vi "Plot menu activation.vi"(7 "BluePlotHandle in":refnum<class "RocketPlotHandle.lvclass">, 8 "error in (no error)":errorcluster, 9 "Coords":T4, 10 "Refs":T5, 11 "MenuRef":refnum<k9>) -> (0 "error out":errorcluster, 1 "Location":T1, 2 "Discard?":bool, 3 "MenuRef":refnum<k9>)   [LabVIEW 2021, in "RocketPlot.lvlib"]
uses:
  RocketPlot.lvlib
  Classes/RocketPlotHandle/RocketPlotHandle.lvclass
  TypeDefs/Plot UI references.ctl
  <userlib>/bjustice/TipStripOOPanel/Classes/TipPanelHandle/TipPanelHandle.lvclass
  TypeDefs/Plot top row.ctl
  <vilib>/Utility/miscctls.llb/LVPoint32TypeDef.ctl
  TypeDefs/Shortcut Location.ctl
  Plot menu activation submenu type v2.ctl
  TypeDefs/Plot axis.ctl
  Plot scale refnum to LUT name.vi
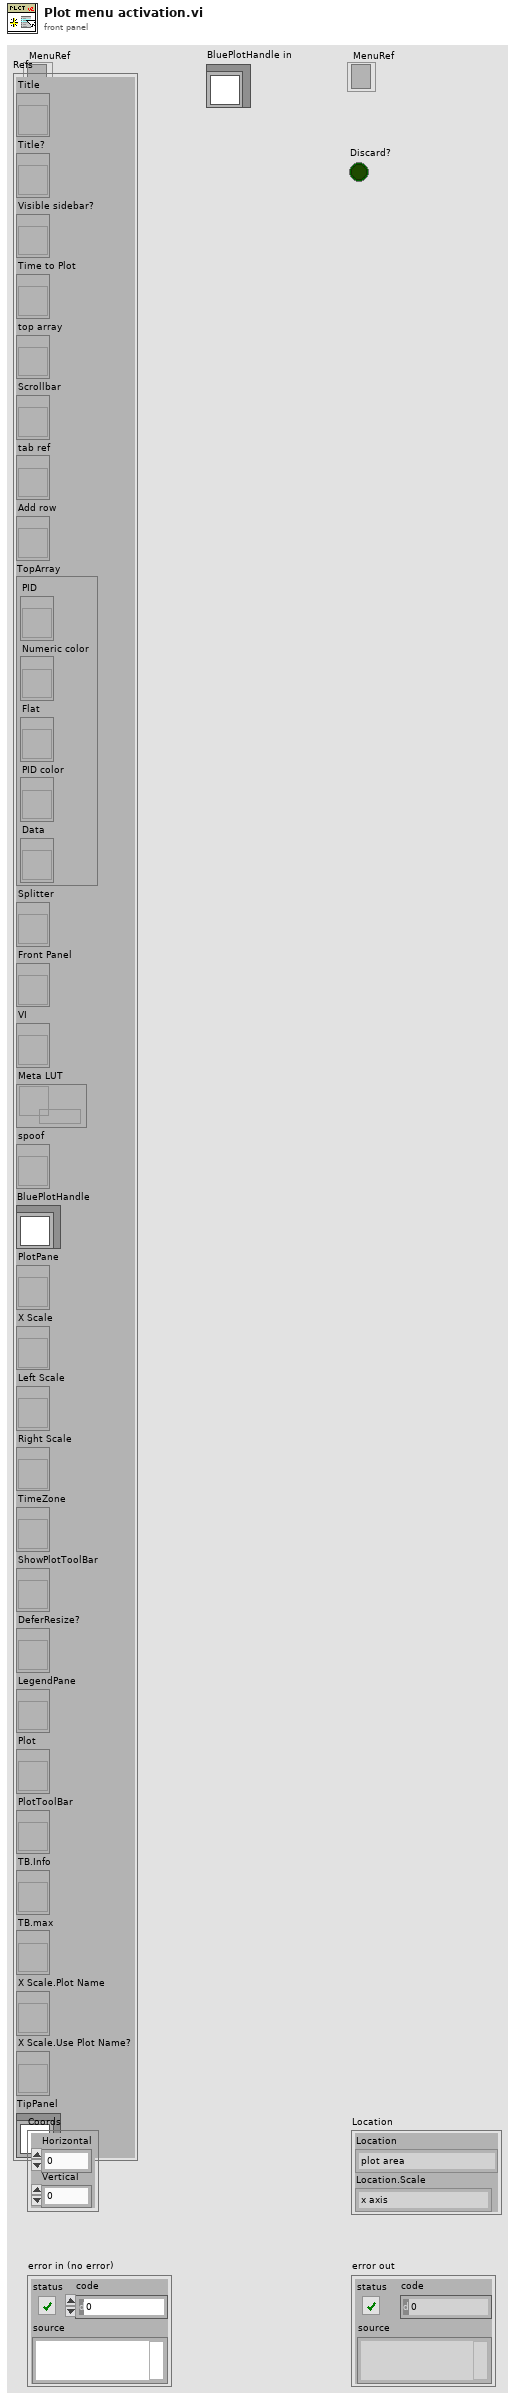
[diagram p1: front panel]
types:
  T1 = typedef "RocketPlot.lvlib/Shortcut Location.ctl" = cluster{"Location":T2, "Location.Scale":T3}
  T2 = typedef "RocketPlot.lvlib/Plot menu activation submenu type v2.ctl" = enum16{"plot area", "plot border", "markers", "scale"}
  T3 = typedef "RocketPlot.lvlib/Plot axis.ctl" = enum16{"x axis", "left axis", "right axis"}
  T4 = typedef "LVPoint32TypeDef.ctl" = cluster{"Horizontal":i32, "Vertical":i32}
  T5 = typedef "RocketPlot.lvlib/Plot UI references.ctl" = cluster{"Title":refnum<vi>, "Title?":refnum<vi>, "Visible sidebar?":refnum<vi>, "Time to Plot":refnum<vi>, "top array":refnum<vi>, "Scrollbar":refnum<vi>, "tab ref":refnum<vi>, "Add row":refnum<vi>, "TopArray":cluster{"PID":refnum<vi>, "Numeric color":refnum<vi>, "Flat":refnum<vi>, "PID color":refnum<vi>, "Data":refnum<vi>}, "Splitter":refnum<vi>, "Front Panel":refnum<vi>, "VI":refnum<vi>, "Meta LUT":refnum<data-value>, "spoof":refnum<vi>, "BluePlotHandle":refnum<class "RocketPlotHandle.lvclass">, "PlotPane":refnum<vi>, "X Scale":refnum<vi>, "Left Scale":refnum<vi>, "Right Scale":refnum<vi>, "TimeZone":refnum<vi>, "ShowPlotToolBar":refnum<vi>, "DeferResize?":refnum<vi>, "LegendPane":refnum<vi>, "Plot":refnum<vi>, "PlotToolBar":refnum<vi>, "TB.Info":refnum<vi>, "TB.max":refnum<vi>, "X Scale.Plot Name":refnum<vi>, "X Scale.Use Plot Name?":refnum<vi>, "TipPanel":refnum<class "TipPanelHandle.lvclass">}
  T6 = typedef "RocketPlot.lvlib/PlatMods.ctl" = cluster{"Shift":bool, "Ctrl":bool, "Alt":bool}
  T7 = typedef "RocketPlot.lvlib/Plot scale meta JSON.ctl" = cluster{"Type":T3, "Grid Colors:Major Color":u32, "Grid Colors:Minor Color":u32, "Style":u8, "Tick Colors:Tick Color":u32, "Tick Colors:Minor Tick Color":u32, "Format String":string, "State":T8, "AxisFocus":refnum<vi>}
  T8 = typedef "RocketPlot.lvlib/Plot scale meta state.ctl" = cluster{"Visible":bool, "Focus":bool, "Multi-Y":bool}
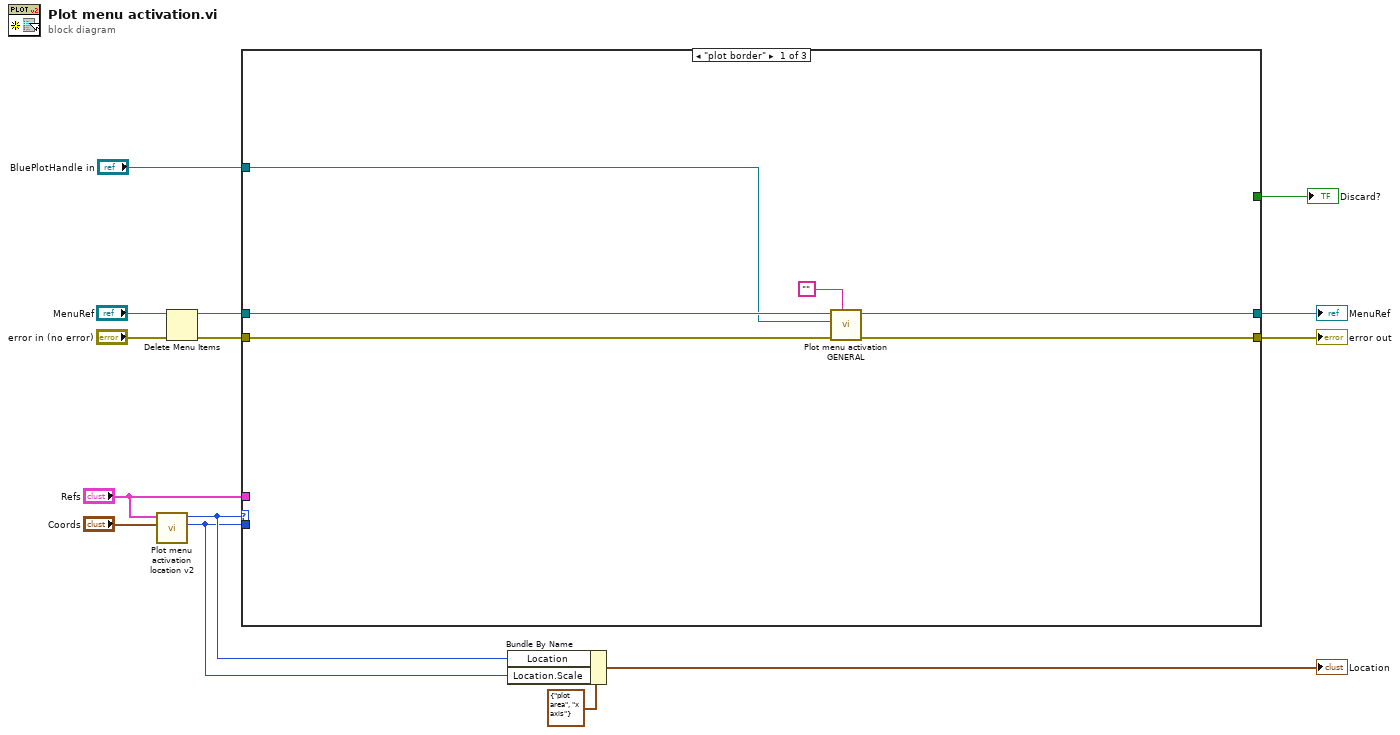
[diagram p0: block diagram]
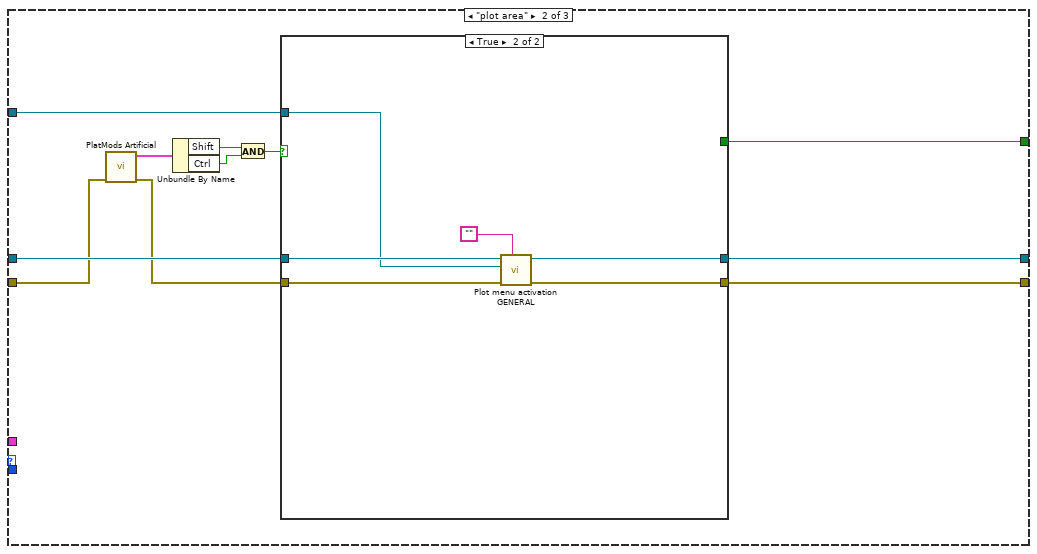
[diagram p2: hidden frame]
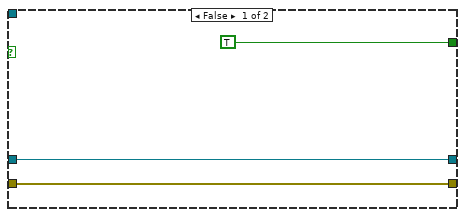
[diagram p3: hidden frame]
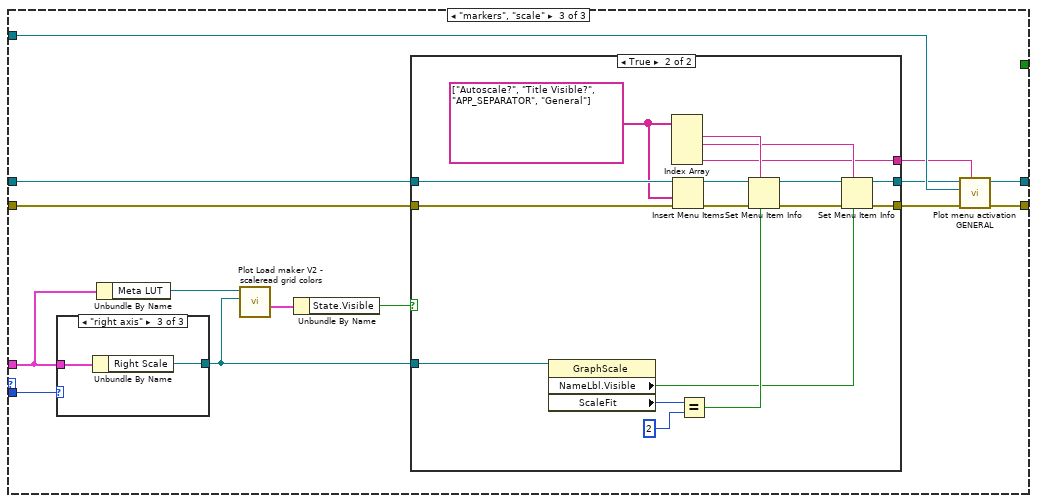
[diagram p4: hidden frame]
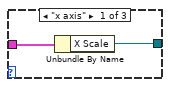
[diagram p6: hidden frame]
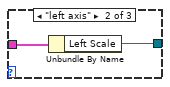
[diagram p7: hidden frame]
diagram:
  n1 = call "Plot menu activation location v2.vi"("Coords"="Coords", "Refs"="Refs") -> ("Location.Scale"=w3:T3, "Location"=w4:T2)  [unwired: 7 in, 1 out]
  n2 = Delete Menu Items(6:"error in (no error)", 9:"MenuRef") -> (0:w9:errorcluster, 3:w10:refnum<k9>)  [unwired: 2 in]
  n3 = case shown="\"plot border\"" w4 {
    tunnel: w3 -> [_ _ w54]
    tunnel: "Refs" -> [_ _ w45]
    tunnel: w10 -> [w18 w30 w53]
    tunnel: w9 -> [w20 w25 w52]
    tunnel: [w19 w31 w50] -> w8
    tunnel: "BluePlotHandle in" -> [w17 w29 w49]
    tunnel: [w15 w28 w46] -> w6
    tunnel: [_ w26 _] -> w1
    frame "plot border" {
      n4 = call "Plot menu activation GENERAL.vi"("menu tag"="", "error in (no error)"=w20, "BluePlotHandle in"=w17, "MenuRef"=w18) -> ("error out"=w19:errorcluster, "MenuRef"=w15:refnum<k9>)  [unwired: 6 in]
    }
    frame "plot area" {
      n5 = call "PlatMods Artificial.vi"("error in (no error)"=w25) -> ("error out"=w24:errorcluster, "PlatMods"=w27:T6)  [unwired: 9 in]
      n6 = Unbundle By Name(w27) -> ("Shift"=w23:bool, "Ctrl"=w22:bool)
      n7 = And(x=w23, y=w22) -> (x .and. y?=w21:bool)
      n8 = case shown="True" w21 {
        tunnel: w24 -> [w33 w40]
        tunnel: [w33 w39] -> w31
        tunnel: w30 -> [w34 w38]
        tunnel: w29 -> [_ w37]
        tunnel: [w34 w35] -> w28
        tunnel: [TRUE _] -> w26
        frame False {
        }
        frame True {
          n9 = call "Plot menu activation GENERAL.vi"("menu tag"="", "error in (no error)"=w40, "BluePlotHandle in"=w37, "MenuRef"=w38) -> ("error out"=w39:errorcluster, "MenuRef"=w35:refnum<k9>)  [unwired: 6 in]
        }
      }
    }
    frame "markers", "scale" {
      n10 = case shown="\"right axis\"" w54 {
        tunnel: w45 -> [w75 w77 w79]
        tunnel: [w74 w76 w78] -> w43
        frame "x axis" {
          n11 = Unbundle By Name(w75) -> ("X Scale"=w74:refnum<vi>)
        }
        frame "left axis" {
          n12 = Unbundle By Name(w77) -> ("Left Scale"=w76:refnum<vi>)
        }
        frame "right axis" {
          n13 = Unbundle By Name(w79) -> ("Right Scale"=w78:refnum<vi>)
        }
      }
      n14 = Unbundle By Name(w45) -> ("Meta LUT"=w44:refnum<data-value>)
      n15 = call "Plot Load maker V2 - scaleread grid colors.vi"("Scale reference"=w43, "Meta LUT"=w44) -> ("Scale LUT meta"=w42:T7)  [unwired: 6 in, 3 out]
      n16 = Unbundle By Name(w42) -> ("State.Visible"=w41:bool)
      n17 = case shown="True" w41 {
        tunnel: w53 -> [w56 w73]
        tunnel: w52 -> [w55 w63]
        tunnel: [w55 w60] -> w51
        tunnel: [w56 w59] -> w48
        tunnel: [_ w58] -> w47
        tunnel: w43 -> [_ w57]
        frame False {
        }
        frame True {
          w71 = string[] ["Autoscale?", "Title Visible?", "APP_SEPARATOR", "General"]
          n18 = property class="GraphScale"(reference=w57) -> ("NameLbl.Visible"=w64:bool, "ScaleFit"=w69:u8)  [unwired: 1 in, 2 out]
          n19 = Index Array(array=w71) -> (element #1=w70:string, element #2=w65:string, element #4=w58:string)  [unwired: 4 in, 1 out]
          n20 = Insert Menu Items(6:w63, 7:w71, 9:w73) -> (0:w62:errorcluster, 3:w72:refnum<k9>)  [unwired: 3 in, 1 out]
          n21 = Equal?(x=w69, y=u8 2) -> (x = y?=w67:bool)
          n22 = Set Menu Item Info(6:w67, 7:w70, 8:w62, 11:w72) -> (0:w61:errorcluster, 3:w66:refnum<k9>)  [unwired: 3 in]
          n23 = Set Menu Item Info(6:w64, 7:w65, 8:w61, 11:w66) -> (0:w60:errorcluster, 3:w59:refnum<k9>)  [unwired: 3 in]
        }
      }
      n24 = call "Plot menu activation GENERAL.vi"("menu tag"=w47, "error in (no error)"=w51, "BluePlotHandle in"=w49, "MenuRef"=w48) -> ("error out"=w50:errorcluster, "MenuRef"=w46:refnum<k9>)  [unwired: 6 in]
    }
  }
  "error out" <- w8
  "MenuRef" <- w6
  "Discard?" <- w1
  n25 = Bundle By Name(cluster=T1 {"Location"=enum."plot area", "Location.Scale"=enum."x axis"} ("Cluster"), "Location"=w4, "Location.Scale"=w3) -> (→"Location":T1)
